vi "calculateXY.vi"(0 "q1":dbl, 1 "q2":dbl, 2 "length 1":dbl, 3 "length 2":dbl) -> (5 "x1 graph (2nd arm)":dbl, 6 "y1 graph (2nd arm)":dbl, 7 "x1 (1st arm)":dbl, 8 "y1 (1st arm)":dbl, 9 "x1 (2nd arm)":dbl, 10 "y1 (2nd arm)":dbl)   [LabVIEW 2023]
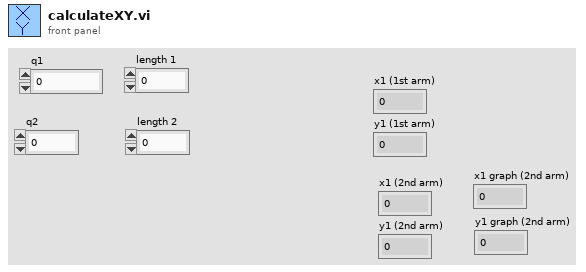
[diagram p1: front panel]
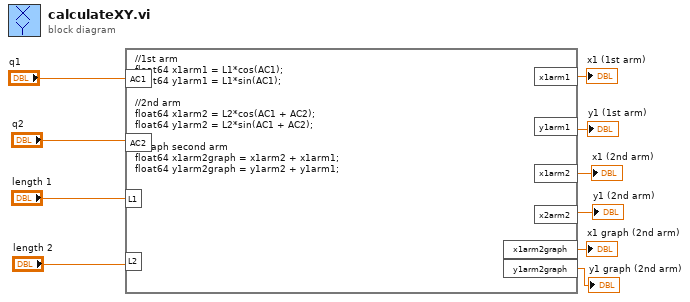
[diagram p0: block diagram]
diagram:
  n1 = formula code="//1st arm\nfloat64 x1arm1 = L1*cos(AC1);\nfloat64 y1arm1 = L1*sin(AC1);\n\n//2nd arm\nfloat64 x1arm2 = L2*cos(AC1 + AC2);\nfloat64 y1arm2 = L2*sin(AC1 + AC2);\n\n//graph second arm\nfloat64 x1arm2graph = x1arm2 + x1arm1;\nfloat64 y1arm2graph = y1arm2 + y1arm1;"("AC1"="q1", "AC2"="q2", "L1"="length 1", "L2"="length 2") -> ("x1arm1"=→"x1 (1st arm)":dbl, "y1arm1"=→"y1 (1st arm)":dbl, "x1arm2"=→"x1 (2nd arm)":dbl, "x2arm2"=→"y1 (2nd arm)":dbl, "x1arm2graph"=→"x1 graph (2nd arm)":dbl, "y1arm2graph"=→"y1 graph (2nd arm)":dbl)
